vi "_Select values for chosen axes.vi"(2 "Queried axes":string[](array[string]), 3 "Values":dbl[](array[numeric]) format="%.6f", 4 "Axes subset":string[](array[string]), 6 "Bool. Values":bool[](array[boolean]), 7 "String values":string[](array[string])) -> (14 "Values subset":dbl[](array[numeric]) format="%.6f", 15 "Bool. Values subset":bool[](array[boolean]), 16 "String values subset":string[](array[string]))   [LabVIEW 2012]
doc: "This VI returns only values for the given axes subset.\n\nValid for Analog systems, C-702, C-843, C-843.PM, C-848, C-865, C-880, C-880K005, E-710, E-761, Mercury"
panel:
  # "This vi returns only values for the given axes subset."
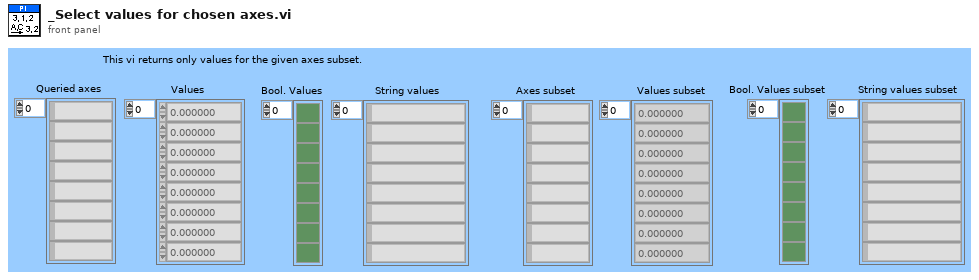
[diagram p1: front panel]
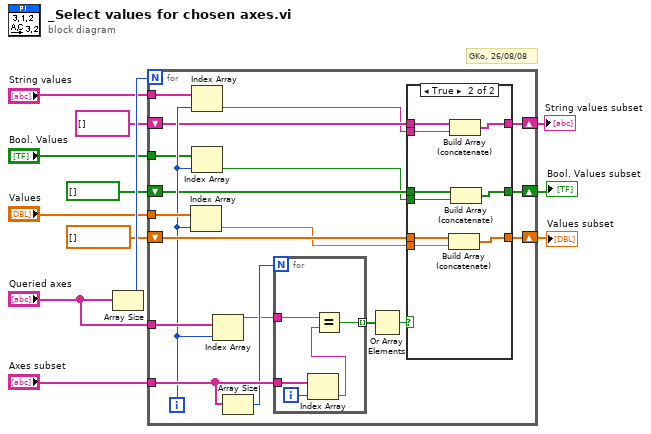
[diagram p0: block diagram]
diagram:
  # "GKo, 26/08/08"
  n1 = Array Size(array="Queried axes") -> (size(s)=w12:i32)
  n2 = for {
    N: w12 -> [_]
    shift-right: [w26] -> w11
    shift-left: dbl[] [] -> [w25]
    tunnel: "Queried axes" -> [w31]
    tunnel: "Axes subset" -> [w30]
    tunnel: "Values" -> [w24]
    tunnel: "String values" -> [w20]
    tunnel: "Bool. Values" -> [w19]
    shift-right: [w16] -> w2
    shift-left: string[] [] -> [w17]
    shift-right: [w15] -> w1
    shift-left: bool[] [] -> [w18]
    i -> [w21]
    n3 = Index Array(array=w24, index=w21) -> (element=w23:dbl)
    n4 = Index Array(array=w20, index=w21) -> (element=w13:string)
    n5 = Index Array(array=w19, index=w21) -> (element=w14:bool)
    n6 = Index Array(array=w31, index=w21) -> (element=w22:string)
    n7 = Array Size(array=w30) -> (size(s)=w29:i32)
    n8 = for {
      N: w29 -> [_]
      tunnel: w22 -> [w44]
      tunnel: w30 -> [w48]
      tunnel: [w45] -> w28 mode=indexing
      i -> [w47]
      n9 = Index Array(array=w48, index=w47) -> (element=w46:string)
      n10 = Equal?(x=w44, y=w46) -> (x = y?=w45:bool)
    }
    n11 = Or Array Elements(Boolean array=w28) -> (logical OR=w27:bool)
    n12 = case shown="True" w27 {
      tunnel: [w34 w43] -> w26
      tunnel: w25 -> [w34 w42]
      tunnel: w23 -> [_ w41]
      tunnel: w18 -> [w32 w40]
      tunnel: w17 -> [w33 w39]
      tunnel: [w33 w38] -> w16
      tunnel: [w32 w37] -> w15
      tunnel: w14 -> [_ w36]
      tunnel: w13 -> [_ w35]
      frame False {
      }
      frame True {
        n13 = Build Array (concatenate)(w42, w41) -> (w43:dbl[])
        n14 = Build Array (concatenate)(w39, w35) -> (w38:string[])
        n15 = Build Array (concatenate)(w40, w36) -> (w37:bool[])
      }
    }
  }
  "Values subset" <- w11
  "Bool. Values subset" <- w1
  "String values subset" <- w2
